vi "Step Update Test Steps 4.0 to 4.1.vi"(8 "error in (no error)":errorcluster, 11 "Connection Refnum":T1) -> (0 "error out":errorcluster, 3 "Connection Refnum Out":T1)   [LabVIEW 2011]
uses:
  www/tests/Get Datasheets From Test Step.vi
  www/tests/Get Test Parameters From Test Step.vi
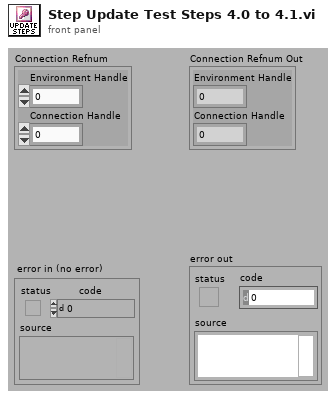
[diagram p1: front panel]
types:
  T1 = cluster{"Environment Handle":i32, "Connection Handle":i32}
  T2 = typedef "Step Record.ctl" = cluster{"ixStep":i32, "sxSequenceId":string, "sxTestId":string, "iIndex":i32, "iRepeat":i32, "iQuickMode":i32, "sTag":string, "sDatasheetsCSV":string, "bConfiguration":string}
  T3 = typedef "Connection Refnum.ctl" = cluster{"Environment Handle":i32, "Connection Handle":i32}
  T4 = typedef "Test Datasheets v1.0-4.0.ctl" = cluster{"Datasheet to Generate":i32, "Print Datasheets":bool}[]
  T5 = typedef "Template Record.ctl" = cluster{"ixTemplate":i32, "sxTemplateId":string, "sDescription":string, "sCreator":string, "tCreationDate":timestamp, "sModifier":string, "tModifiedDate":timestamp, "sType":string, "sStyle":string, "sFormat":string, "dWidth":dbl, "dHeight":dbl, "sFilename":string, "sScript":string, "sLayout":string, "sEditor":string, "sStyleProcess":string}
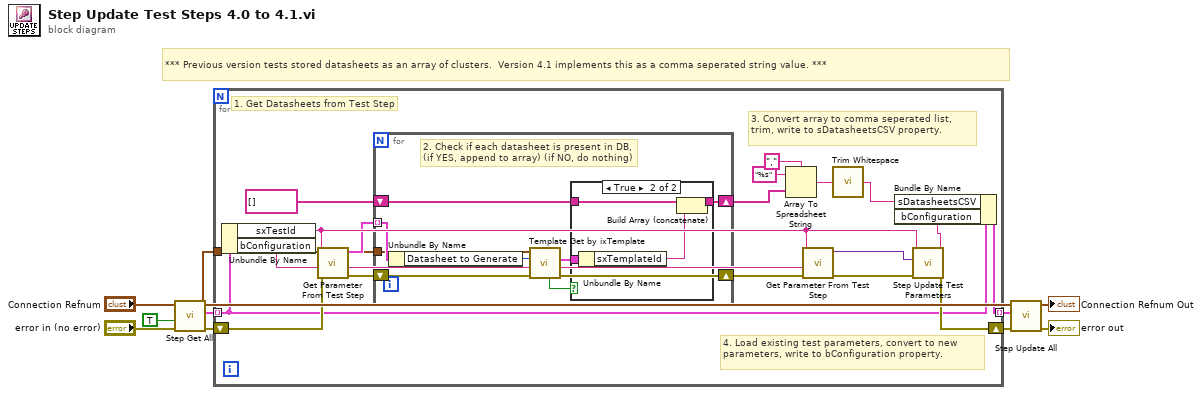
[diagram p0: block diagram]
diagram:
  # "*** Previous version tests stored datasheets as an array of clusters.  Version 4.1 implements this as a comma seperated string value. ***"
  n1 = call "Step Get All.vi"("error in (no error)"="error in (no error)", "All Steps? (f)"=TRUE, "Connection Refnum"="Connection Refnum") -> ("error out"=w9:errorcluster, "Sequence Steps"=w8:T2[], "Connection Refnum"=w1:T3)  [unwired: 1 in, 5 out]
  n2 = for {
    shift-right: [w28] -> w7
    shift-left: w9 -> [w29]
    tunnel: w8 -> [w27] mode=indexing
    tunnel: [w25] -> w6 mode=indexing
    tunnel: w1 -> [w17]
    # "4. Load existing test parameters, convert to new parameters, write to bConfiguration property."
    # "3. Convert array to comma seperated list, trim, write to sDatasheetsCSV property."
    # "1. Get Datasheets from Test Step"
    n3 = Unbundle By Name(w27) -> ("sxTestId"=w23:string, "bConfiguration"=w24:string)
    n4 = call-poly "Get Parameter From Test Step.vi"("error in (no error)"=w29, "Test Configuration (\"\")"=w24, "Test_ID (\"\")"=w23) -> ("error out"=w20:errorcluster, "Datasheets"=w18:T4)  [unwired: 7 out]
    n5 = for {
      shift-right: [w36] -> w19
      shift-left: w20 -> [w38]
      tunnel: w18 -> [w37] mode=indexing
      shift-right: [w31] -> w13
      shift-left: string[] [] -> [w32]
      tunnel: w17 -> [w30]
      # "2. Check if each datasheet is present in DB,\n(if YES, append to array) (if NO, do nothing)"
      n6 = Unbundle By Name(w37) -> ("Datasheet to Generate"=w35:i32)
      n7 = call "Template Get by ixTemplate.vi"("error in (no error)"=w38, "ixTemplate (0)"=w35, "Connection Refnum"=w30) -> ("error out"=w36:errorcluster, "Template Record"=w34:T5, "Data Present"=w33:bool)  [unwired: 6 out]
      n8 = case shown="True" w33 {
        tunnel: w34 -> [_ w43]
        tunnel: w32 -> [w39 w42]
        tunnel: [w39 w41] -> w31
        frame False {
          # "Do not add if the \ntemplate no longer\nexists in the database."
        }
        frame True {
          n9 = Unbundle By Name(w43) -> ("sxTemplateId"=w40:string)
          n10 = Build Array (concatenate)(w42, w40) -> (w41:string[])
        }
      }
    }
    n11 = Array To Spreadsheet String(delimiter (Tab)=",", array=w13, 3:"%s" ("format string")) -> (spreadsheet string=w12:string)
    n12 = call-poly "Get Parameter From Test Step.vi"("error in (no error)"=w19, "Test Configuration (\"\")"=w24, "Test_ID (\"\")"=w23) -> ("error out"=w22:errorcluster, "Test Parameters"=w21:variant)  [unwired: 7 out]
    n13 = call <vilib>:"Trim Whitespace.vi"("string"=w12) -> ("trimmed string"=w11:string)  [unwired: 1 in]
    n14 = call "Step Update Test Parameters.vi"("error in (no error)"=w22, "Test Parameters"=w21, "Test_ID (\"\")"=w23) -> ("error out"=w28:errorcluster, "Parameter String"=w26:string)  [unwired: 1 in, 6 out]
    n15 = Bundle By Name(cluster=w27, "sDatasheetsCSV"=w11, "bConfiguration"=w26) -> (w25:T2)
  }
  n16 = call "Step Update All.vi"("error in (no error)"=w7, "Steps"=w6, "Connection Refnum"=w1) -> ("error out"=→"error out":errorcluster, "Connection Refnum"=→"Connection Refnum Out":T3)  [unwired: 7 out]
